vi "dbc_demo.vi"(0 "DLL类型":u32(ring) items=["ControlCAN", "zlgcan"], 5 "设备类型":u32(ring)=1 items=["PCI5121"=1, "PCI9810"=2, "USBCAN1"=3, "USBCAN2"=4, "PCI9820"=5, "PCI5110"=7, "PC104CAN"=11, "CANETUDP"=12, "PCI9840B"=14, "PC104C2"=15, "PCI9820I"=16, "CANETTCP"=17, "PCIE9221"=24, "PCI5010U"=19, "USBCAN_E_U"=20, "USBCAN_2E_U"=21, "CANalyst-II+"=10021, "PCI5020U"=22, "PCIE9120I"=27, "PCIE9110I"=28, "PCIE9140I"=29, "PCIE_CANFD_100U"=38, "PCIE_CANFD_200U"=39, "PCIE_CANFD_400U"=40, "USBCANFD_200U"=41, "USBCANFD_100U"=42, "云设备"=46], 7 "设备索引":u32, 9 "通道索引":u32, 11 "设备打开状态":bool) -> ()   [LabVIEW 2020]
uses:
  DBCHandle.vi
  DeviceInfo.vi
  bin/LibDBCManager.dll
  RetVal.vi
  LVMessageHandle.vi
  bin/dbc_demo_api.dll
  Signals.vi
  bin/ControlCAN.dll
  VCI_CAN_OBJ_R.vi
  VCI_CAN_OBJ_N.vi
panel:
  out "临时字符串":string
  out "数据日志":string
  in  "DBC信号":i32(listbox)
  in  "加载DBC":bool
  in  "DBC消息":i32(listbox)
  in  "DBC文件路径":path
  in  "发送":bool
  in  "确定修改":bool
  in  "当前信号值：":dbl
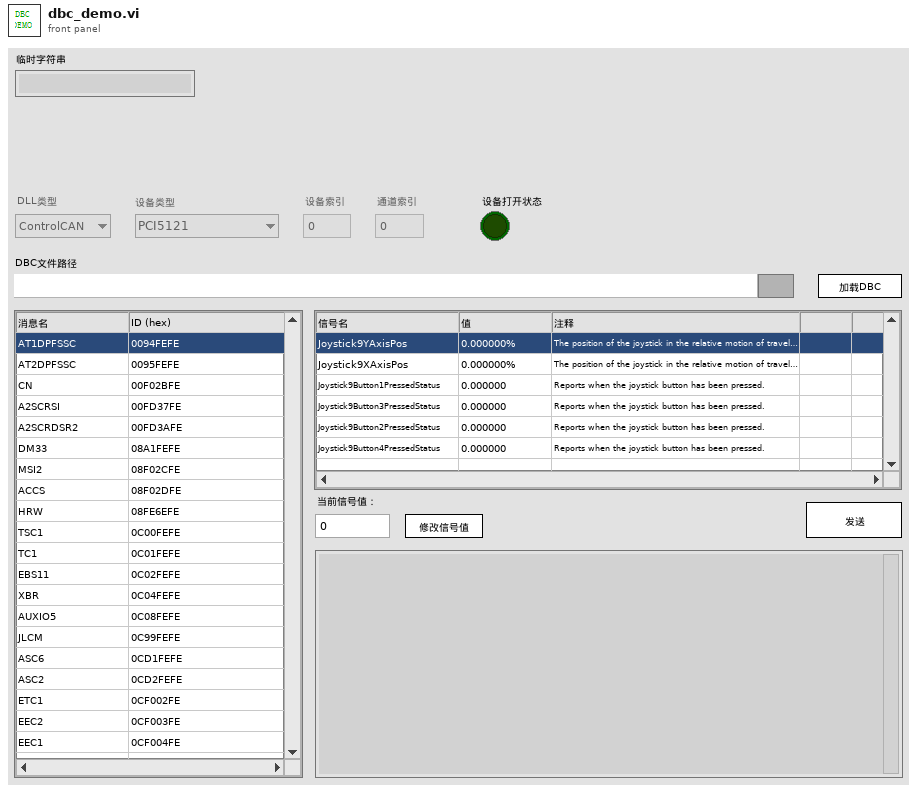
[diagram p1: front panel]
types:
  T1 = cluster{"ID":u32, "TimeStamp":u32, "TimeFlag":u8, "SendType":u8, "RemoteFlag":u8, "ExternFlag":u8, "DataLen":u8, "Data":u8, u8, u8, u8, u8, u8, u8, u8, "Reserved0":u8, "Reserved1":u8, "Reserved2":u8}
  T2 = cluster{"ID":u32, "TimeStamp":u32, "TimeFlag":u8, "SendType":u8, "RemoteFlag":u8, "ExternFlag":u8, "DataLen":u8, "Data":u8, u8, u8, u8, u8, u8, u8, u8, "Reserved0":u8, "Reserved1":u8, "Reserved2":u8}[]
  T3 = cluster{"DLL类型":u32, "设备类型":u32, "设备索引":u32, "CAN通道号":u32}
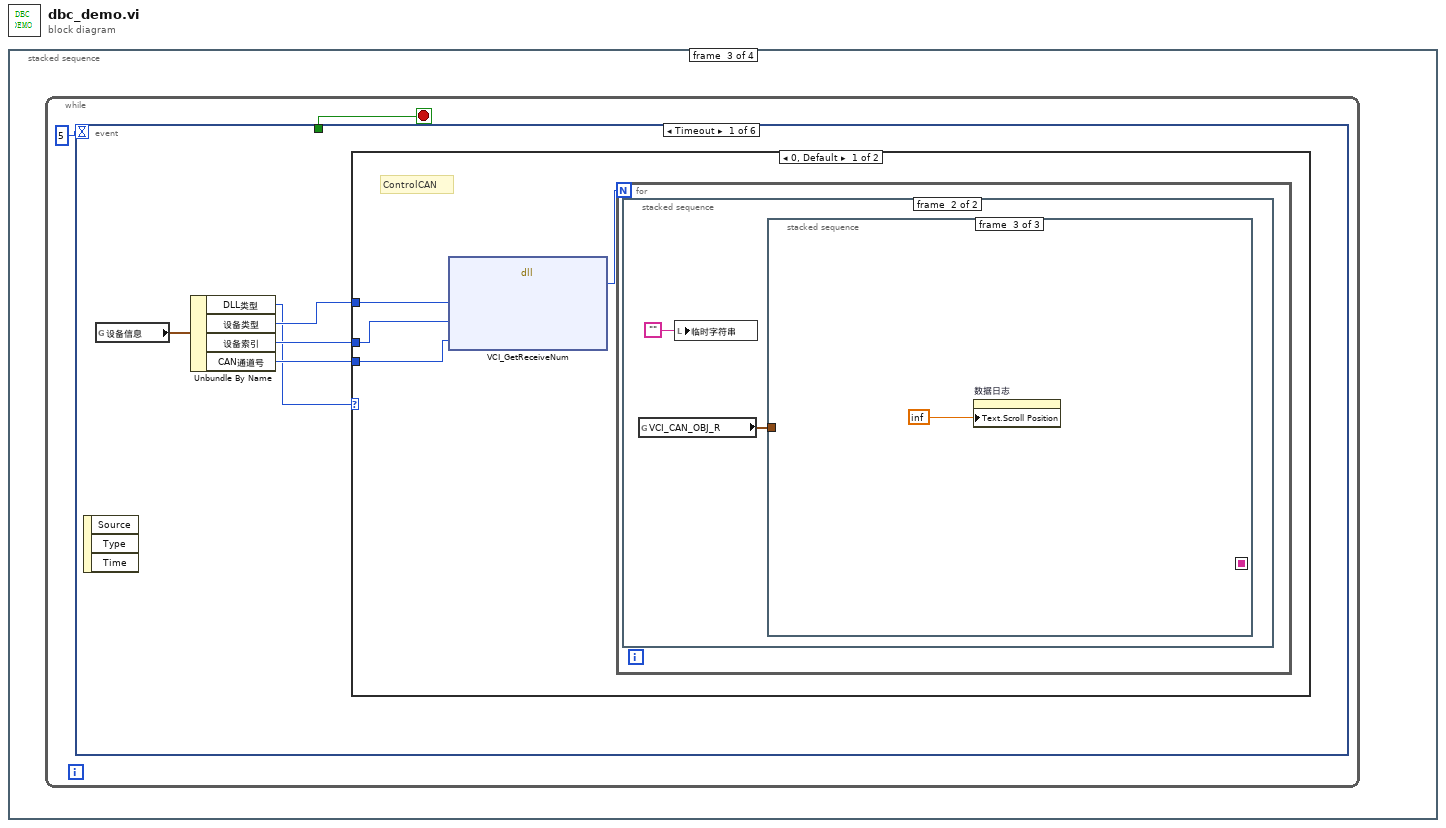
[diagram p0: block diagram]
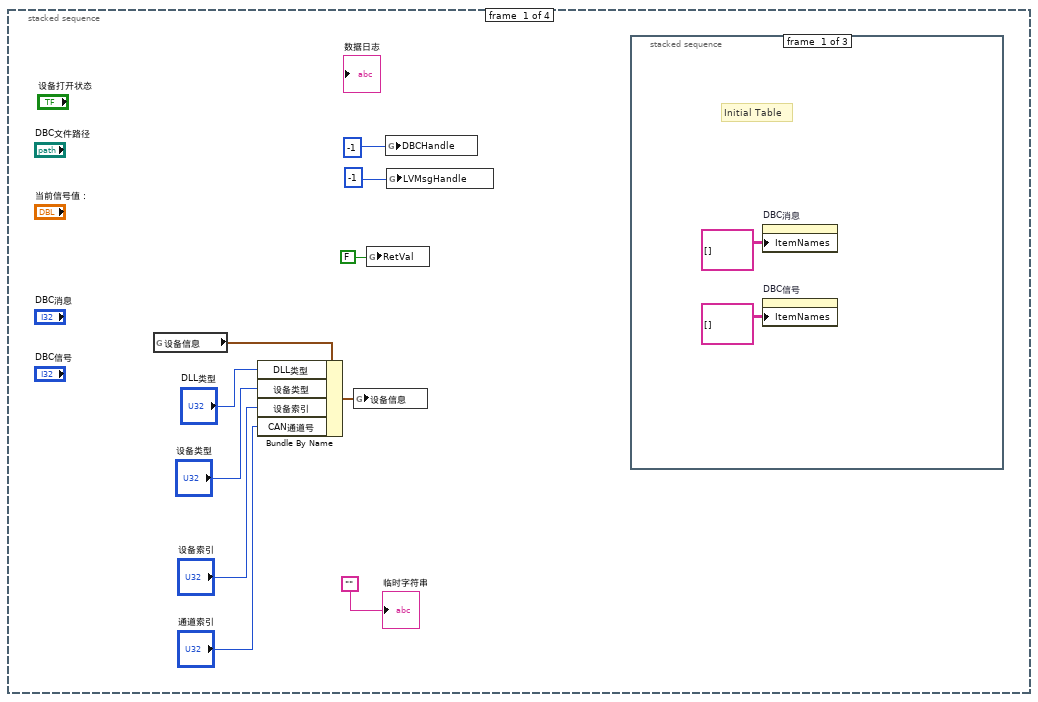
[diagram p2: hidden frame]
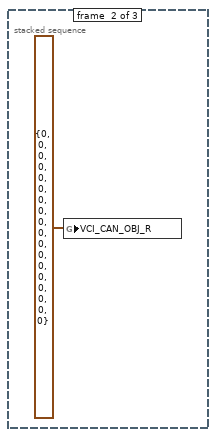
[diagram p3: hidden frame]
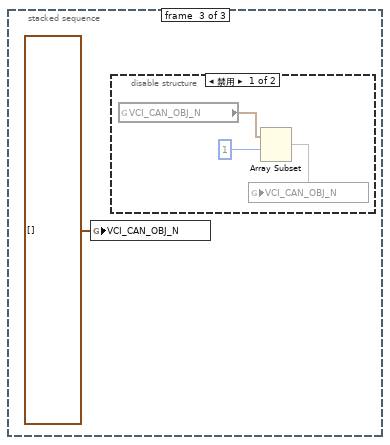
[diagram p4: hidden frame]
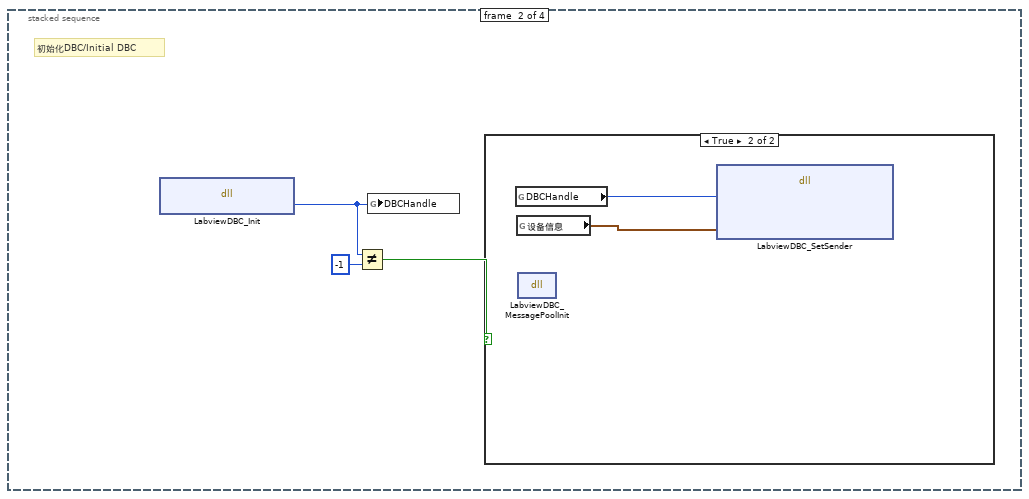
[diagram p6: hidden frame]
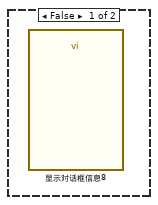
[diagram p7: hidden frame]
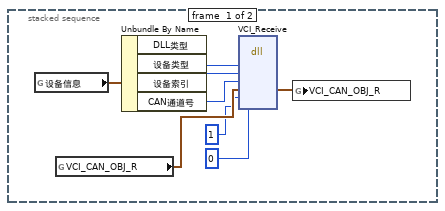
[diagram p8: hidden frame]
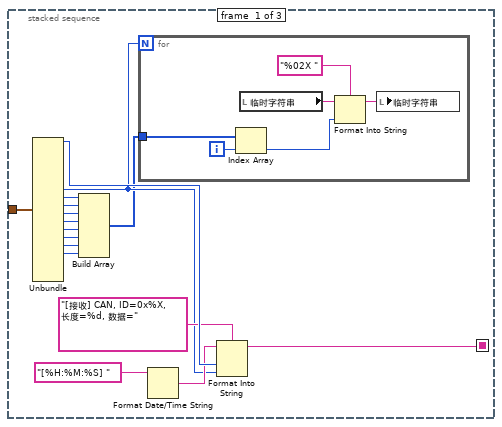
[diagram p9: hidden frame]
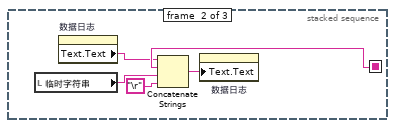
[diagram p10: hidden frame]
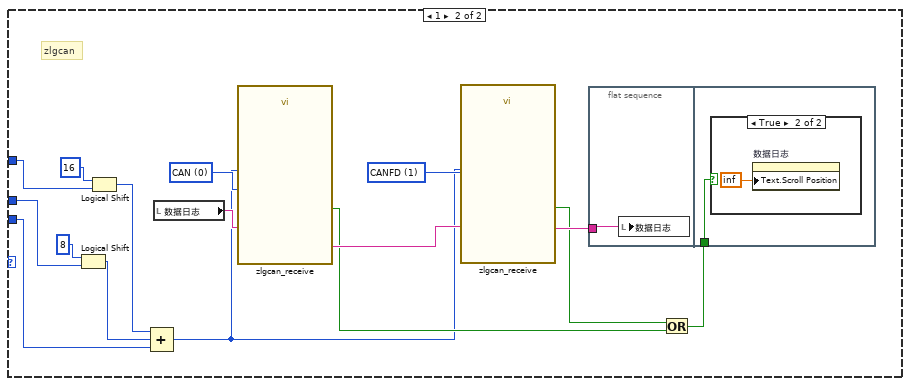
[diagram p11: hidden frame]
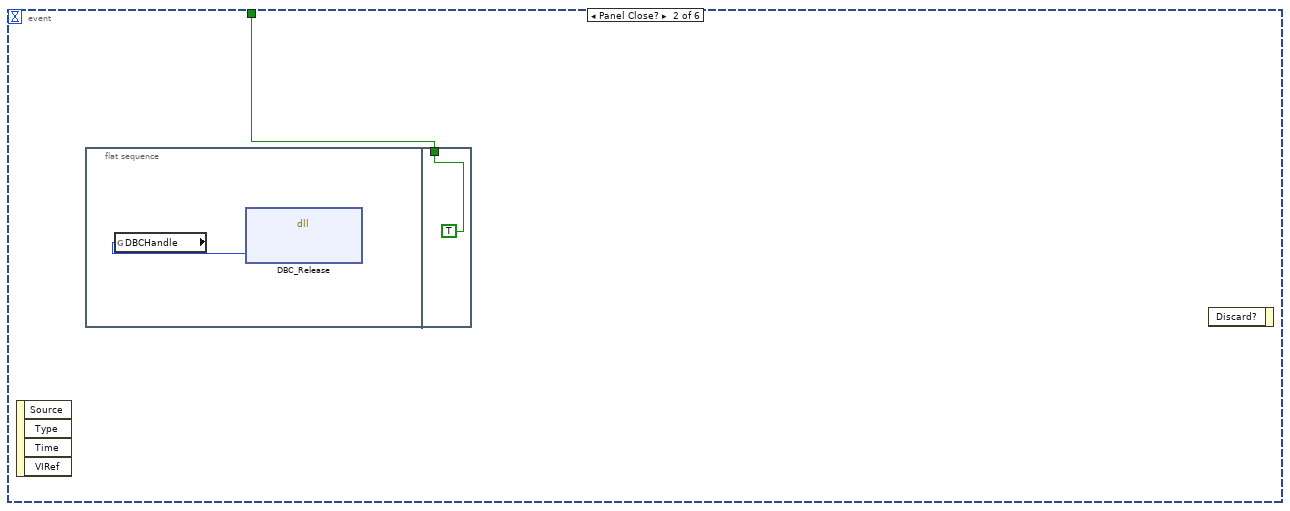
[diagram p13: hidden frame]
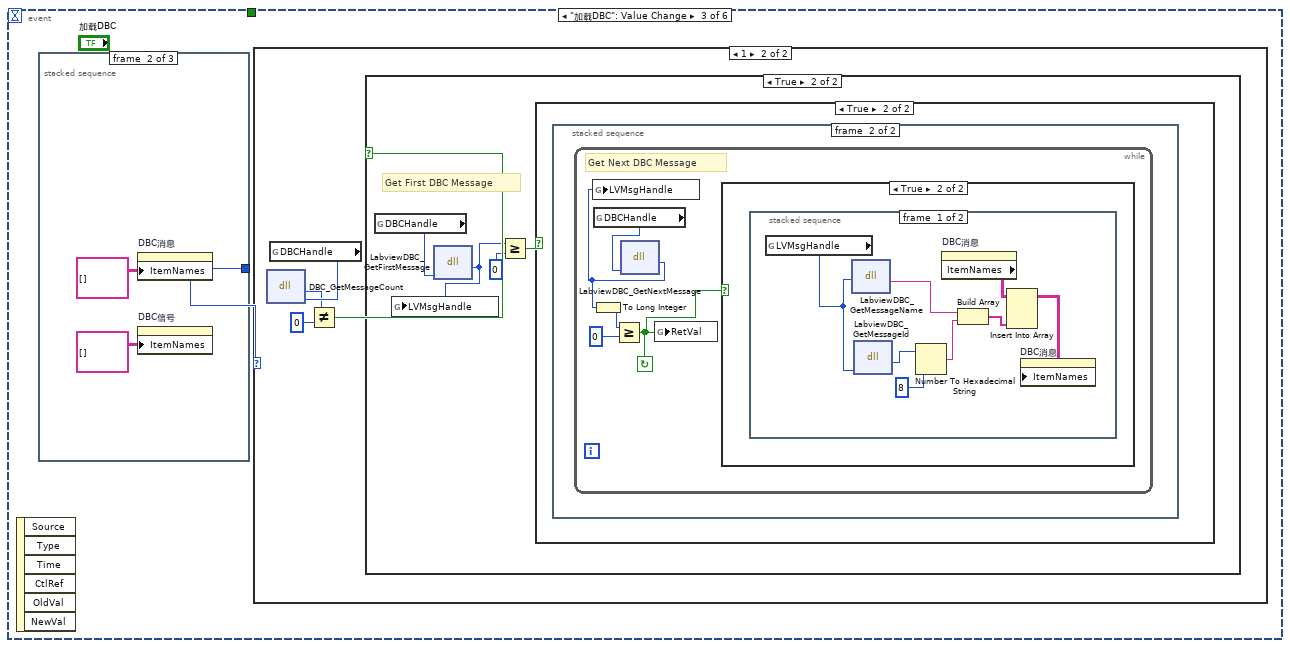
[diagram p14: hidden frame]
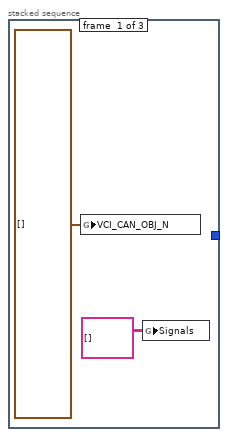
[diagram p15: hidden frame]
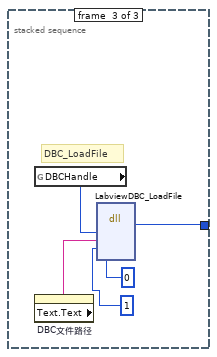
[diagram p16: hidden frame]
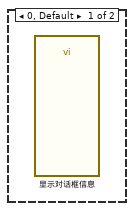
[diagram p17: hidden frame]
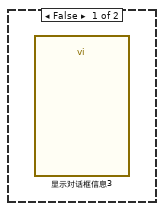
[diagram p18: hidden frame]
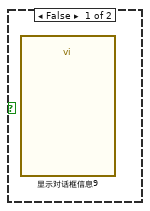
[diagram p19: hidden frame]
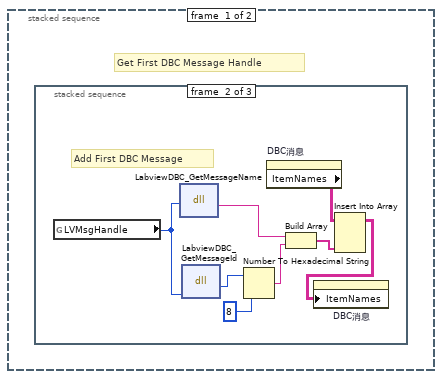
[diagram p20: hidden frame]
diagram:
  n1 = stacked-sequence {
    frame #0 {
      n2 = global read "DeviceInfo.vi" "设备信息"() -> (w9:T3)
      n3 = Bundle By Name(cluster=w9, "DLL类型"="DLL类型", "设备类型"="设备类型", "设备索引"="设备索引", "CAN通道号"="通道索引") -> (w8:T3)
      n4 = global write "DeviceInfo.vi" "设备信息"(w8) -> ()
      n5 = global write "RetVal.vi" "RetVal"(FALSE ("RetVal")) -> ()
      n6 = global write "DBCHandle.vi" "DBCHandle"(-1) -> ()
      n7 = global write "LVMessageHandle.vi" "LVMsgHandle"(-1 ("LVMessageHandle")) -> ()
      n8 = stacked-sequence {
        frame #0 {
          # "Initial Table"
          n9 = property on="DBC消息" class="MCListbox (strict)"("ItemNames"=string[][] [] ("项名")) -> ()  [unwired: 2 in, 2 out]
          n10 = property on="DBC信号" class="MCListbox (strict)"("ItemNames"=string[][] [] ("项名")) -> ()  [unwired: 2 in, 2 out]
        }
        frame #1 {
          n11 = global write "VCI_CAN_OBJ_R.vi" "VCI_CAN_OBJ_R"(T1 {"ID"=0, "TimeStamp"=0, "TimeFlag"=0, "SendType"=0, "RemoteFlag"=0, "ExternFlag"=0, "DataLen"=0, "Data"=0, 0, 0, 0, 0, 0, 0, 0, "Reserved0"=0, "Reserved1"=0, "Reserved2"=0} ("VCI_CAN_OBJ_R")) -> ()
        }
        frame #2 {
          n12 = global write "VCI_CAN_OBJ_N.vi" "VCI_CAN_OBJ_N"(T2 [] ("VCI_CAN_OBJ_N")) -> ()
          n13 = disable-structure shown="禁用" {
            frame Disabled {
              n14 = global read "VCI_CAN_OBJ_N.vi" "VCI_CAN_OBJ_N"() -> (w16:T2)
              n15 = Array Subset(array=w16, index=1 ("索引")) -> (w15:T2)  [unwired: 1 in]
              n16 = global write "VCI_CAN_OBJ_N.vi" "VCI_CAN_OBJ_N"(w15) -> ()
            }
            frame Enabled {
            }
          }
        }
      }
      "临时字符串" <- ""
    }
    frame #1 {
      # "初始化DBC/Initial DBC"
      n17 = dll-call lib="E:/Project/CANMaster/LabView/ControlCAN_labview/bin/dbc_demo_api.dll" fn="LabviewDBC_Init"() -> ("DBCHandle"=w20:u32)  [unwired: 3 in, 2 out]
      n18 = Not Equal?(x=w20, y=-1) -> (x != y?=w18:bool)
      n19 = global write "DBCHandle.vi" "DBCHandle"(w20) -> ()
      n20 = case shown="True" w18 {
        frame False {
          n21 = call "显示对话框信息8"() -> ()  [unwired: 10 in, 2 out]
        }
        frame True {
          n22 = global read "DBCHandle.vi" "DBCHandle"() -> (w21:u32)
          n23 = global read "DeviceInfo.vi" "设备信息"() -> (w22:T3)
          n24 = dll-call lib="E:/Project/CANMaster/LabView/ControlCAN_labview/bin/dbc_demo_api.dll" fn="LabviewDBC_MessagePoolInit"() -> ()  [unwired: 4 in, 2 out]
          n25 = dll-call lib="E:/Project/CANMaster/LabView/ControlCAN_labview/bin/dbc_demo_api.dll" fn="LabviewDBC_SetSender"("DBCHandle"=w21, "ctx"=w22) -> ()  [unwired: 6 in, 2 out]
        }
      }
    }
    frame #2 {
      n26 = while {
        stop <- w23 stop-if-true
        n27 = event shown="[0] Timeout" {
          selector: _ -> [_ _ _ _ _ _]
          dyn-events: _ -> [_ _ _ _ _ _]
          timeout: 5 -> [_ _ _ _ _ _]
          tunnel: [_ w91 _ _ _ _] -> w23
          event Timeout {
            n28 = event-data() -> ()  [unwired: 1 in, 3 out]
            n29 = global read "DeviceInfo.vi" "设备信息"() -> (w29:T3)
            n30 = Unbundle By Name(w29) -> ("DLL类型"=w25:u32, "设备类型"=w28:u32, "设备索引"=w26:u32, "CAN通道号"=w27:u32)
            n31 = case shown="0, Default" w25 {
              tunnel: w28 -> [w33 w74]
              tunnel: w27 -> [w31 w72]
              tunnel: w26 -> [w30 w79]
              frame 0, Default {
                # "ControlCAN"
                n32 = dll-call lib="E:/Project/CANMaster/LabView/ControlCAN_labview/bin/ControlCAN.dll" fn="VCI_GetReceiveNum"("DeviceType"=w33, "DeviceInd"=w30, "CANInd"=w31) -> ("返回类型"=w32:u64)  [unwired: 6 in, 2 out]
                n33 = for {
                  N: w32 -> [_]
                  n34 = stacked-sequence {
                    frame #0 {
                      n35 = global read "DeviceInfo.vi" "设备信息"() -> (w37:T3)
                      n36 = global read "VCI_CAN_OBJ_R.vi" "VCI_CAN_OBJ_R"() -> (w41:T1)
                      n37 = Unbundle By Name(w37) -> ("设备类型"=w38:u32, "设备索引"=w39:u32, "CAN通道号"=w40:u32)  [unwired: 1 out]
                      n38 = dll-call lib="E:/Project/CANMaster/LabView/ControlCAN_labview/bin/ControlCAN.dll" fn="VCI_Receive"("DeviceType"=w38, "DeviceInd"=w39, "CANInd"=w40, "pReceive"=w41, "Len"=u64 1, "WaitTime"=0 ("timeout")) -> ("pReceive"=w34:T1)  [unwired: 8 in, 3 out]
                      n39 = global write "VCI_CAN_OBJ_R.vi" "VCI_CAN_OBJ_R"(w34) -> ()
                    }
                    frame #1 {
                      n40 = global read "VCI_CAN_OBJ_R.vi" "VCI_CAN_OBJ_R"() -> (w43:T1)
                      n41 = local write "临时字符串"("") -> ()
                      n42 = stacked-sequence {
                        seq-local: [w59 _ _] -> [_ w68 _]
                        tunnel: w43 -> [w44 _ _]
                        frame #0 {
                          n43 = Unbundle(w44) -> ("ID"=w58:u32, "DataLen"=w54:u8, "Data"=w46:u8, w47:u8, w48:u8, w49:u8, w50:u8, w51:u8, w52:u8, w53:u8)  [unwired: 8 out]
                          n44 = Build Array(w46, w47, w48, w49, w50, w51, w52, w53) -> (w45:u8[])
                          n45 = for {
                            N: w54 -> [_]
                            tunnel: w45 -> [w60]
                            i -> [w65]
                            n46 = Index Array(array=w60, index=w65) -> (element=w63:u8)
                            n47 = local read "临时字符串"() -> (w62:string)
                            n48 = Format Into String(format string="%02X " ("格式字符串"), initial string=w62, w63) -> (resulting string=w61:string)  [unwired: 1 in, 1 out]
                            n49 = local write "临时字符串"(w61) -> ()
                          }
                          n50 = Format Date/Time String(time format string (%c)="[%H:%M:%S] " ("时间格式字符串(%c)")) -> (date/time string=w55:string)  [unwired: 2 in]
                          n51 = Format Into String(format string="[接收] CAN, ID=0x%X, 长度=%d, 数据=" ("格式字符串"), initial string=w55, w58, w54) -> (resulting string=w59:string)  [unwired: 1 in, 1 out]
                        }
                        frame #1 {
                          n52 = local read "临时字符串"() -> (w70:string)
                          n53 = property on="数据日志" class="Str"() -> ("Text.Text"=w67:string)  [unwired: 2 in, 2 out]
                          n54 = Concatenate Strings(w67, w68, w70, "\r") -> (w66:string)
                          n55 = property on="数据日志" class="Str"("Text.Text"=w66) -> ()  [unwired: 2 in, 2 out]
                        }
                        frame #2 {
                          n56 = property on="数据日志" class="Str"("Text.Scroll Position"=inf) -> ()  [unwired: 2 in, 2 out]
                        }
                      }
                    }
                  }
                }
              }
              frame 1 {
                w85 = u16 1 items=["CAN", "CANFD"] ("协议")
                w86 = u16 0 items=["CAN", "CANFD"] ("协议")
                # "zlgcan"
                n57 = Logical Shift(y=i16 8, x=w79) -> (x << y=w76:u32)
                n58 = Logical Shift(y=i16 16, x=w74) -> (x << y=w73:u32)
                n59 = Compound Arithmetic op=ADD(w73, w76, w72) -> (w75:u32)
                n60 = local read "数据日志"() -> (w87:string)
                n61 = call "zlgcan_receive.vi"("输入字符串"=w87, "协议"=w86, "通道句柄"=w75) -> ("输出字符串"=w83:string, "结果"=w82:bool)
                n62 = call "zlgcan_receive.vi"("输入字符串"=w83, "协议"=w85, "通道句柄"=w75) -> ("输出字符串"=w84:string, "结果"=w81:bool)
                n63 = flat-sequence {
                  tunnel: w84 -> [w88]
                  tunnel: w80 -> [w89]
                  frame #0 {
                    n64 = local write "数据日志"(w88) -> ()
                  }
                  frame #1 {
                    n65 = case shown="True" w89 {
                      frame False {
                      }
                      frame True {
                        n66 = property on="数据日志" class="Str"("Text.Scroll Position"=inf) -> ()  [unwired: 2 in, 2 out]
                      }
                    }
                  }
                }
                n67 = Or(x=w81, y=w82) -> (x .or. y?=w80:bool)
              }
            }
          }
          event Panel Close? {
            n68 = event-data() -> ()  [unwired: 1 in, 4 out]
            n69 = flat-sequence {
              tunnel: [TRUE] -> w91
              frame #0 {
                n70 = global read "DBCHandle.vi" "DBCHandle"() -> (w92:u32)
                n71 = dll-call lib="E:/Project/CANMaster/LabView/ControlCAN_labview/bin/LibDBCManager.dll" fn="DBC_Release"("DBCHandle"=w92) -> ()  [unwired: 5 in, 2 out]
              }
              frame #1 {
              }
            }
            n72 = event-data() -> ()  [unwired: 2 in, 1 out]
          }
          event "加载DBC": Value Change {
            n73 = event-data() -> ()  [unwired: 1 in, 6 out]
            n74 = stacked-sequence {
              tunnel: [_ _ w99] -> w94
              frame #0 {
                n75 = global write "VCI_CAN_OBJ_N.vi" "VCI_CAN_OBJ_N"(T2 [] ("VCI_CAN_OBJ_N")) -> ()
                n76 = global write "Signals.vi" "Signals"(string[][] [] ("Signals")) -> ()
              }
              frame #1 {
                n77 = property on="DBC消息" class="MCListbox (strict)"("ItemNames"=string[][] [] ("项名")) -> ()  [unwired: 2 in, 2 out]
                n78 = property on="DBC信号" class="MCListbox (strict)"("ItemNames"=string[][] [] ("项名")) -> ()  [unwired: 2 in, 2 out]
              }
              frame #2 {
                # "DBC_LoadFile"
                n79 = global read "DBCHandle.vi" "DBCHandle"() -> (w102:u32)
                n80 = property on="DBC文件路径" class="Path"() -> ("Text.Text"=w103:string)  [unwired: 2 in, 2 out]
                n81 = dll-call lib="E:/Project/CANMaster/LabView/ControlCAN_labview/bin/dbc_demo_api.dll" fn="LabviewDBC_LoadFile"("DBCHandle"=w102, "strPath"=w103, "type"=u8 1, "merge"=u8 0) -> ("返回类型"=w99:u8)  [unwired: 7 in, 2 out]
              }
            }
            n82 = case shown="1" w94 {
              frame 0, Default {
                n83 = call "显示对话框信息"() -> ()  [unwired: 10 in, 2 out]
              }
              frame 1 {
                n84 = global read "DBCHandle.vi" "DBCHandle"() -> (w107:u32)
                n85 = dll-call lib="E:/Project/CANMaster/LabView/ControlCAN_labview/bin/LibDBCManager.dll" fn="DBC_GetMessageCount"("DBCHandle"=w107) -> ("返回类型"=w104:u32)  [unwired: 4 in, 2 out]
                n86 = Not Equal?(x=w104, y=u32 0) -> (x != y?=w106:bool)
                n87 = case shown="True" w106 {
                  frame False {
                    n88 = call "显示对话框信息3"() -> ()  [unwired: 10 in, 2 out]
                  }
                  frame True {
                    # "Get First DBC Message"
                    n89 = global read "DBCHandle.vi" "DBCHandle"() -> (w111:u32)
                    n90 = dll-call lib="E:/Project/CANMaster/LabView/ControlCAN_labview/bin/dbc_demo_api.dll" fn="LabviewDBC_GetFirstMessage"("DBCHandle"=w111) -> ("hMsg"=w109:u32)  [unwired: 4 in, 2 out]
                    n91 = global write "LVMessageHandle.vi" "LVMsgHandle"(w109) -> ()
                    n92 = Greater Or Equal?(x=w109, y=u32 0) -> (x >= y?=w110:bool)
                    n93 = case shown="True" w110 {
                      frame False {
                        n94 = call "显示对话框信息9"() -> ()  [unwired: 10 in, 2 out]
                      }
                      frame True {
                        n95 = stacked-sequence {
                          frame #0 {
                            # "Get First DBC Message Handle"
                            n96 = stacked-sequence {
                              frame #0 {
                                # "Clear DBC Message Table"
                                n97 = property on="DBC消息" class="MCListbox (strict)"("ItemNames"=string[][] [] ("项名")) -> ()  [unwired: 2 in, 2 out]
                              }
                              frame #1 {
                                # "Add First DBC Message"
                                n98 = global read "LVMessageHandle.vi" "LVMsgHandle"() -> (w117:u32)
                                n99 = dll-call lib="E:/Project/CANMaster/LabView/ControlCAN_labview/bin/dbc_demo_api.dll" fn="LabviewDBC_GetMessageName"("hMsg"=w117) -> ("返回类型"=w114:string)  [unwired: 4 in, 2 out]
                                n100 = dll-call lib="E:/Project/CANMaster/LabView/ControlCAN_labview/bin/dbc_demo_api.dll" fn="LabviewDBC_GetMessageId"("hMsg"=w117) -> ("返回类型"=w115:u32)  [unwired: 4 in, 2 out]
                                n101 = Number To Hexadecimal String(1:i16 8 ("宽度(-)"), 2:w115) -> (0:w116:string)
                                n102 = property on="DBC消息" class="MCListbox (strict)"() -> ("ItemNames"=w118:string[][])  [unwired: 2 in, 2 out]
                                n103 = Build Array(w114, w116) -> (w119:string[])
                                n104 = Insert Into Array(array=w118, new element=w119) -> (w120:string[][])  [unwired: 2 in]
                                n105 = property on="DBC消息" class="MCListbox (strict)"("ItemNames"=w120) -> ()  [unwired: 2 in, 2 out]
                              }
                              frame #2 {
                                # "Relese Message"
                                n106 = global read "LVMessageHandle.vi" "LVMsgHandle"() -> (w121:u32)
                                n107 = dll-call lib="E:/Project/CANMaster/LabView/ControlCAN_labview/bin/dbc_demo_api.dll" fn="LabviewDBC_FreeMessage"("hMsg"=w121) -> ()  [unwired: 5 in, 2 out]
                              }
                            }
                          }
                          frame #1 {
                            n108 = while {
                              stop <- w124 continue-if-true
                              # "Get Next DBC Message"
                              n109 = global read "DBCHandle.vi" "DBCHandle"() -> (w126:u32)
                              n110 = dll-call lib="E:/Project/CANMaster/LabView/ControlCAN_labview/bin/dbc_demo_api.dll" fn="LabviewDBC_GetNextMessage"("DBCHandle"=w126) -> ("hMsgHandle"=w123:u32)  [unwired: 4 in, 2 out]
                              n111 = global write "LVMessageHandle.vi" "LVMsgHandle"(w123) -> ()
                              n112 = To Long Integer(number=w123) -> (32bit integer=w122:i32)
                              n113 = Greater Or Equal?(x=w122, y=i8 0) -> (x >= y?=w124:bool)
                              n114 = global write "RetVal.vi" "RetVal"(w124) -> ()
                              n115 = case shown="True" w124 {
                                frame False {
                                }
                                frame True {
                                n116 = stacked-sequence {
                                frame #0 {
                                n117 = global read "LVMessageHandle.vi" "LVMsgHandle"() -> (w133:u32)
                                n118 = dll-call lib="E:/Project/CANMaster/LabView/ControlCAN_labview/bin/dbc_demo_api.dll" fn="LabviewDBC_GetMessageName"("hMsg"=w133) -> ("返回类型"=w130:string)  [unwired: 4 in, 2 out]
                                n119 = dll-call lib="E:/Project/CANMaster/LabView/ControlCAN_labview/bin/dbc_demo_api.dll" fn="LabviewDBC_GetMessageId"("hMsg"=w133) -> ("返回类型"=w131:u32)  [unwired: 4 in, 2 out]
                                n120 = Number To Hexadecimal String(1:i16 8 ("宽度(-)"), 2:w131) -> (0:w132:string)
                                n121 = property on="DBC消息" class="MCListbox (strict)"() -> ("ItemNames"=w128:string[][])  [unwired: 2 in, 2 out]
                                n122 = Build Array(w130, w132) -> (w134:string[])
                                n123 = Insert Into Array(array=w128, new element=w134) -> (w127:string[][])  [unwired: 2 in]
                                n124 = property on="DBC消息" class="MCListbox (strict)"("ItemNames"=w127) -> ()  [unwired: 2 in, 2 out]
                                }
                                frame #1 {
                                # "Relese Message"
                                n125 = global read "LVMessageHandle.vi" "LVMsgHandle"() -> (w135:u32)
                                n126 = dll-call lib="E:/Project/CANMaster/LabView/ControlCAN_labview/bin/dbc_demo_api.dll" fn="LabviewDBC_FreeMessage"("hMsg"=w135) -> ()  [unwired: 5 in, 2 out]
                                }
                                }
                                }
                              }
                            }
                          }
                        }
                      }
                    }
                  }
                }
              }
            }
          }
          event "DBC消息": Value Change {
            n127 = event-data() -> ()  [unwired: 1 in, 6 out]
            n128 = property on="DBC消息" class="MCListbox (strict)"() -> ("ItemNames"=w146:string[][])  [unwired: 2 in, 2 out]
            n129 = property on="DBC消息" class="MCListbox (strict)"() -> ("FocusRow"=w145:i32)  [unwired: 2 in, 2 out]
            n130 = Index Array(array=w146, index (row)=w145) -> (element=w144:string[])  [unwired: 1 in]
            n131 = Index Array(array=w144, index=1 ("索引")) -> (element=w142:string)
            n132 = global read "DBCHandle.vi" "DBCHandle"() -> (w140:u32)
            n133 = Hexadecimal String To Number(string=w142) -> (number=w141:u32)  [unwired: 2 in, 1 out]
            n134 = dll-call lib="E:/Project/CANMaster/LabView/ControlCAN_labview/bin/dbc_demo_api.dll" fn="LabviewDBC_GetMessageById"("hDBC"=w140, "nID"=w141) -> ("hMsg"=w137:u32)  [unwired: 5 in, 2 out]
            n135 = To Long Integer(number=w137) -> (32bit integer=w139:i32)
            n136 = global write "LVMessageHandle.vi" "LVMsgHandle"(w137) -> ()
            n137 = Not Equal?(x=w139, y=-1) -> (x != y?=w136:bool)
            n138 = case shown="True" w136 {
              frame False {
              }
              frame True {
                n139 = stacked-sequence {
                  frame #0 {
                    n140 = property on="DBC信号" class="MCListbox (strict)"("ItemNames"=string[][] [] ("项名")) -> ()  [unwired: 2 in, 2 out]
                    n141 = global write "Signals.vi" "Signals"(string[][] [] ("Signals")) -> ()
                  }
                  frame #1 {
                    (unwired) -1 ("y")
                    n142 = global read "LVMessageHandle.vi" "LVMsgHandle"() -> (w152:u32)
                    n143 = dll-call lib="E:/Project/CANMaster/LabView/ControlCAN_labview/bin/dbc_demo_api.dll" fn="LabviewDBC_GetMessageSignalNum"("hMsg"=w152) -> ("nSignalCount"=w149:i32)  [unwired: 4 in, 2 out]
                    n144 = Not Equal?(x=w149, y=-1) -> (x != y?=w151:bool)
                    n145 = case shown="True" w151 {
                      tunnel: w149 -> [_ w153]
                      frame False {
                      }
                      frame True {
                        n146 = for {
                          N: w153 -> [_]
                          i -> [w157]
                          n147 = global read "LVMessageHandle.vi" "LVMsgHandle"() -> (w161:u32)
                          n148 = property on="DBC信号" class="MCListbox (strict)"() -> ("ItemNames"=w159:string[][])  [unwired: 2 in, 2 out]
                          n149 = call "Signal2List.vi"("nSignalIndex"=w157, "hMsg"=w161) -> ("Value and Unit"=w155:string[], "Signal List"=w160:string[])  [unwired: 2 in]
                          n150 = global read "Signals.vi" "Signals"() -> (w156:string[][])
                          n151 = Insert Into Array(array=w156, new element=w155) -> (w154:string[][])  [unwired: 2 in]
                          n152 = Insert Into Array(array=w159, new element=w160) -> (w158:string[][])  [unwired: 2 in]
                          n153 = global write "Signals.vi" "Signals"(w154) -> ()
                          n154 = property on="DBC信号" class="MCListbox (strict)"("ItemNames"=w158) -> ()  [unwired: 2 in, 2 out]
                        }
                      }
                    }
                  }
                  frame #2 {
                    # "Relese Message"
                    n155 = global read "LVMessageHandle.vi" "LVMsgHandle"() -> (w162:u32)
                    n156 = dll-call lib="E:/Project/CANMaster/LabView/ControlCAN_labview/bin/dbc_demo_api.dll" fn="LabviewDBC_FreeMessage"("hMsg"=w162) -> ()  [unwired: 5 in, 2 out]
                  }
                }
              }
            }
          }
          event "确定修改": Value Change {
            n157 = event-data() -> ()  [unwired: 1 in, 6 out]
            n158 = stacked-sequence {
              frame #0 {
                n159 = global read "Signals.vi" "Signals"() -> (w163:string[][])
                n160 = property on="DBC信号" class="MCListbox (strict)"() -> ("FocusRow"=w164:i32)  [unwired: 2 in, 2 out]
                n161 = in-place {
                  n162 = in-place-array #1(w163, w164, 0) -> ()  [unwired: 1 out]
                  n163 = local read "当前信号值："() -> (w168:dbl)
                  n164 = Number To Fractional String(number=w168) -> (F-format string=w167:string)  [unwired: 3 in]
                  n165 = in-place-array #1(w167) -> (w166:string[][])  [unwired: 2 out]
                }
                n166 = global write "Signals.vi" "Signals"(w166) -> ()
              }
              frame #1 {
                n167 = property on="DBC信号" class="MCListbox (strict)"() -> ("ItemNames"=w170:string[][])  [unwired: 2 in, 2 out]
                n168 = property on="DBC信号" class="MCListbox (strict)"() -> ("FocusRow"=w171:i32)  [unwired: 2 in, 2 out]
                n169 = in-place {
                  n170 = in-place-array #2(w170, w171, 1) -> ()  [unwired: 1 out]
                  n171 = global read "Signals.vi" "Signals"() -> (w176:string[][])
                  n172 = property on="DBC信号" class="MCListbox (strict)"() -> ("FocusRow"=w175:i32)  [unwired: 2 in, 2 out]
                  n173 = Index Array(array=w176, index (row)=w175) -> (element=w173:string[])  [unwired: 1 in]
                  n174 = Concatenate Strings(w173) -> (w174:string)
                  n175 = in-place-array #2(w174) -> (w172:string[][])  [unwired: 2 out]
                }
                n176 = property on="DBC信号" class="MCListbox (strict)"("ItemNames"=w172) -> ()  [unwired: 2 in, 2 out]
              }
            }
          }
          event "发送": Value Change {
            n177 = event-data() -> ()  [unwired: 1 in, 6 out]
            n178 = stacked-sequence {
              frame #0 {
                n179 = property on="DBC消息" class="MCListbox (strict)"() -> ("ItemNames"=w178:string[][])  [unwired: 2 in, 2 out]
                n180 = local read "DBC消息"() -> (w177:i32)
                n181 = Index Array(array=w178, index (row)=w177) -> (element=w180:string[])  [unwired: 1 in]
                n182 = Index Array(array=w180, index=1 ("索引")) -> (element=w181:string)
                n183 = global read "DBCHandle.vi" "DBCHandle"() -> (w183:u32)
                n184 = Hexadecimal String To Number(string=w181) -> (number=w182:u32)  [unwired: 2 in, 1 out]
                n185 = dll-call lib="E:/Project/CANMaster/LabView/ControlCAN_labview/bin/dbc_demo_api.dll" fn="LabviewDBC_GetMessageById"("hDBC"=w183, "nID"=w182) -> ("hMsg"=w184:u32)  [unwired: 5 in, 2 out]
                n186 = global write "LVMessageHandle.vi" "LVMsgHandle"(w184) -> ()
              }
              frame #1 {
                n187 = global read "LVMessageHandle.vi" "LVMsgHandle"() -> (w186:u32)
                n188 = dll-call lib="E:/Project/CANMaster/LabView/ControlCAN_labview/bin/dbc_demo_api.dll" fn="LabviewDBC_GetMessageSignalNum"("hMsg"=w186) -> ("nSignalCount"=w185:i32)  [unwired: 4 in, 2 out]
                n189 = for {
                  N: w185 -> [_]
                  i -> [w191]
                  n190 = global read "Signals.vi" "Signals"() -> (w192:string[][])
                  n191 = global read "LVMessageHandle.vi" "LVMsgHandle"() -> (w193:u32)
                  n192 = Index Array(array=w192, index (row)=w191) -> (element=w190:string[])  [unwired: 1 in]
                  n193 = Index Array(array=w190, index=0 ("索引")) -> (element=w188:string)
                  n194 = Fract/Exp String To Number(string=w188) -> (number=w187:dbl)  [unwired: 3 in, 1 out]
                  n195 = dll-call lib="E:/Project/CANMaster/LabView/ControlCAN_labview/bin/dbc_demo_api.dll" fn="LabviewDBC_SetSignalValueByMessage"("hMsg"=w193, "nSignalIndex"=w191, "nValue"=w187) -> ()  [unwired: 7 in, 2 out]
                }
              }
              frame #2 {
                n196 = global read "LVMessageHandle.vi" "LVMsgHandle"() -> (w198:u32)
                n197 = global read "DBCHandle.vi" "DBCHandle"() -> (w199:u32)
                n198 = dll-call lib="E:/Project/CANMaster/LabView/ControlCAN_labview/bin/dbc_demo_api.dll" fn="LabviewDBC_Send"("hDBC"=w199, "hMsg"=w198) -> ("返回类型"=w197:u8)  [unwired: 5 in, 2 out]
                n199 = Not Equal?(x=w197, y=u8 0) -> (x != y?=w194:bool)
                n200 = case shown="True" w194 {
                  tunnel: ["[发送] 数据发送失败！" "[发送] 数据发送成功。"] -> w195
                  frame False {
                  }
                  frame True {
                  }
                }
                n201 = stacked-sequence {
                  tunnel: w195 -> [w203 _]
                  frame #0 {
                    n202 = local read "数据日志"() -> (w205:string)
                    n203 = Format Date/Time String(time format string (%c)="[%H:%M:%S] " ("时间格式字符串(%c)")) -> (date/time string=w201:string)  [unwired: 2 in]
                    n204 = Concatenate Strings(w205, w201, w203, "\r") -> (w202:string)
                    n205 = local write "数据日志"(w202) -> ()
                  }
                  frame #1 {
                    n206 = property on="数据日志" class="Str"("Text.Scroll Position"=inf) -> ()  [unwired: 2 in, 2 out]
                  }
                }
              }
              frame #3 {
                # "Relese Message"
                n207 = global read "LVMessageHandle.vi" "LVMsgHandle"() -> (w209:u32)
                n208 = dll-call lib="E:/Project/CANMaster/LabView/ControlCAN_labview/bin/dbc_demo_api.dll" fn="LabviewDBC_FreeMessage"("hMsg"=w209) -> ()  [unwired: 5 in, 2 out]
              }
            }
          }
        }
      }
    }
    frame #3 {
      n209 = flat-sequence {
        frame #0 {
          n210 = global read "DBCHandle.vi" "DBCHandle"() -> (w212:u32)
          n211 = Not Equal?(x=-1, y=w212) -> (x != y?=w211:bool)
          n212 = case shown="True" w211 {
            tunnel: w212 -> [_ w213]
            frame False {
            }
            frame True {
              n213 = dll-call lib="E:/Project/CANMaster/LabView/ControlCAN_labview/bin/dbc_demo_api.dll" fn="LabviewDBC_Release"("DBCHandle"=w213) -> ()  [unwired: 5 in, 2 out]
            }
          }
        }
      }
    }
  }
